vi "FM_RTL-SDR_RX - V4-Script1.vi"() -> ()   [LabVIEW 2013]
uses:
  <vilib>/sound2/lvsound2.llb/Sound Data Format.ctl
  <vilib>/Analysis/2dsp.llb/Rational Resample (single channel, DBL).vi
  <vilib>/sound2/lvsound2.llb/Sound Output Write (DBL Single).vi
  <instrlib>/rtlsdr/rtlsdr.lvlib
  <vilib>/Analysis/NI_AALPro.lvlib
panel:
  in  "Device index":u32
  out "Samples Acquired":u32
  out "# elements in queue":i32
  out "DevRefnum":u64
  out "XY Graph":cluster{dbl[], dbl[]}(graph)
  out "error out":errorcluster
  in  "sound format":T1={"sample rate (S/s)"=44100.0, "number of channels"=1, "bits per sample"=16}
  in  "stop":bool
  in  "Center frequency":u32=104300000
  in  "IQ rate":u32=286650
  out "error out":errorcluster
  # "FM Receiver"
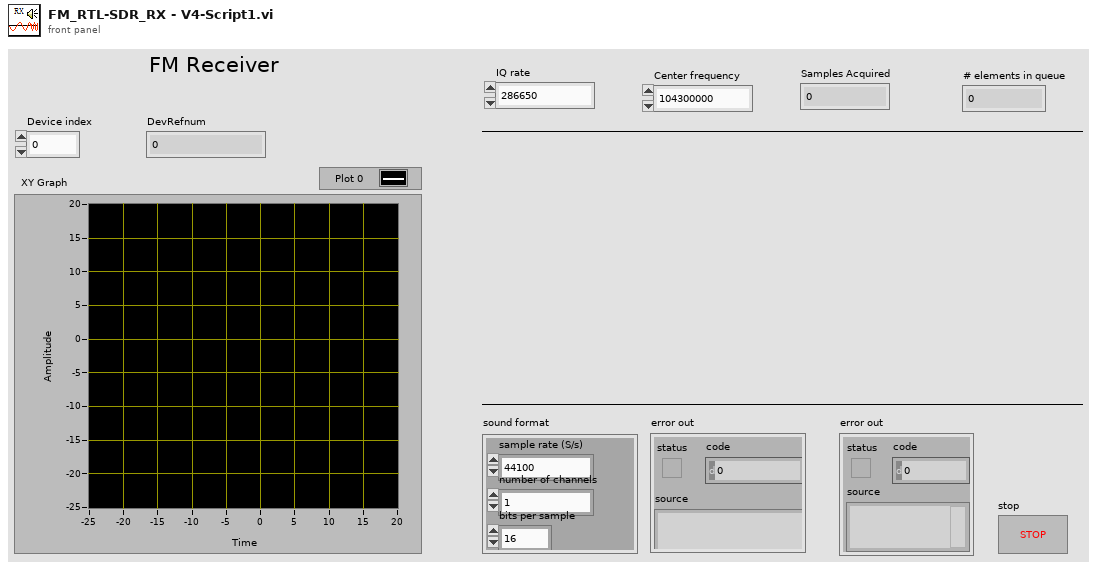
[diagram p1: front panel]
types:
  T1 = typedef "Sound Data Format.ctl" = cluster{"sample rate (S/s)":dbl, "number of channels":i32, "bits per sample":i32}
  T2 = typedef "Sound Output Task ID.ctl" = u32
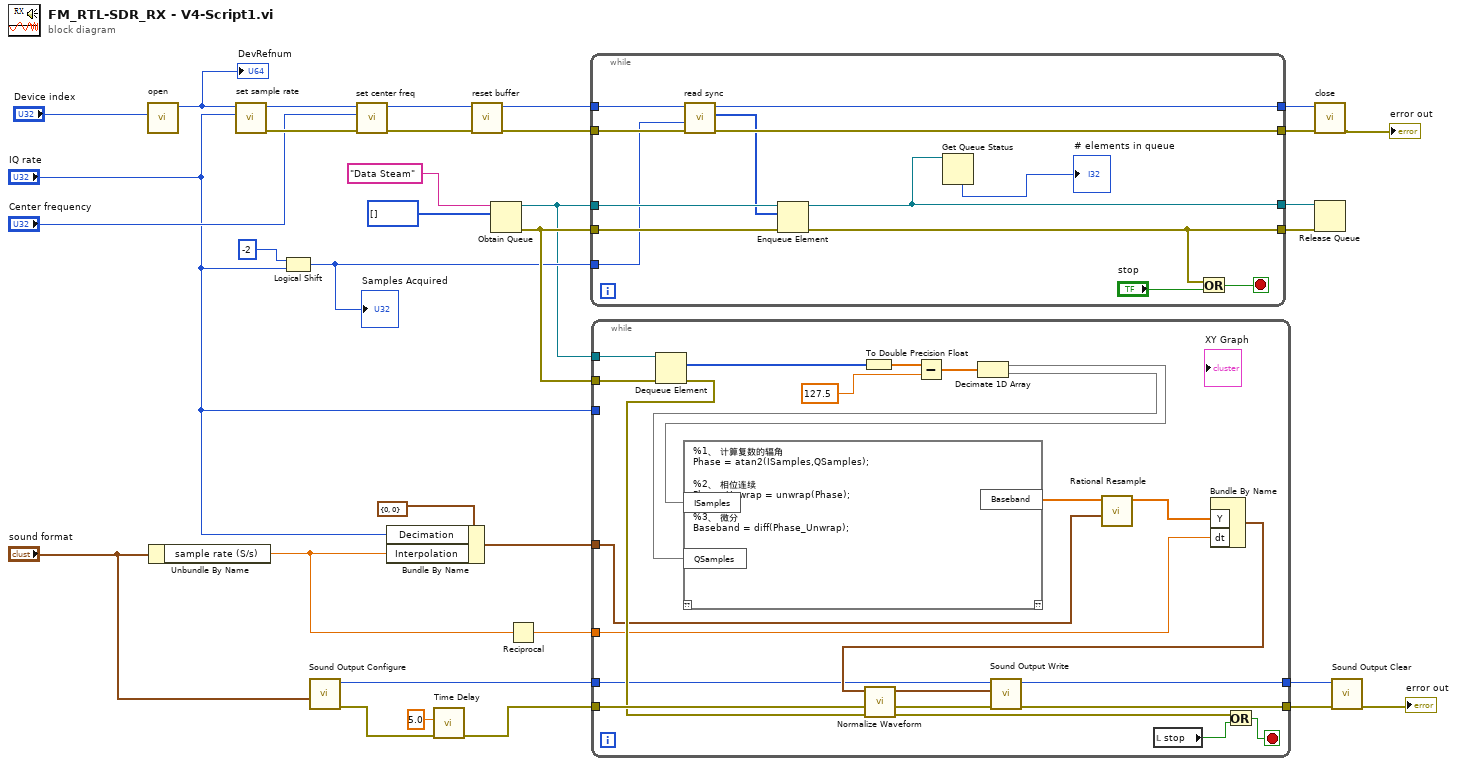
[diagram p0: block diagram]
diagram:
  n1 = call <instrlib>:"open.vi"("index"="Device index") -> ("DevRefnum"=w26:u64)  [unwired: 9 in, 1 out]
  "DevRefnum" <- w26
  n2 = Unbundle By Name("sound format") -> ("sample rate (S/s)"=w1:dbl)
  n3 = call <instrlib>:"set sample rate.vi"("rate"="IQ rate", "DevRefnum"=w26) -> ("error out"=w28:errorcluster, "DevRefnum"=w30:u64)  [unwired: 7 in, 1 out]
  n4 = Logical Shift(y=i16 -2, x="IQ rate") -> (x << y=w4:u32)
  "Samples Acquired" <- w4
  n5 = call <vilib>:"Sound Output Configure.vi"("sound format"="sound format") -> ("error out"=w8:errorcluster, "task ID"=w18:T2)  [unwired: 9 in]
  n6 = call <instrlib>:"set center freq.vi"("error in (no error)"=w28, "freq"="Center frequency", "DevRefnum"=w30) -> ("error out"=w27:errorcluster, "DevRefnum"=w29:u64)  [unwired: 6 in, 1 out]
  n7 = Bundle By Name(cluster=cluster{"Interpolation":i32, "Decimation":i32} {"Interpolation"=0, "Decimation"=0}, "Decimation"="IQ rate", "Interpolation"=w1) -> (w10:cluster{"Interpolation":i32, "Decimation":i32})
  n8 = call "Time Delay"("error in (no error)"=w8, "Delay Time (s)"=5.0) -> ("error out"=w9:errorcluster)  [unwired: 9 in]
  n9 = call <instrlib>:"reset buffer.vi"("error in (no error)"=w27, "DevRefnum"=w29) -> ("error out"=w23:errorcluster, "DevRefnum"=w24:u64)  [unwired: 8 in]
  n10 = Obtain Queue(name (unnamed)="Data Steam", element data type=u8[] [] ("buf 2")) -> (queue out=w3:refnum<queue>, error out=w5:errorcluster)  [unwired: 3 in, 1 out]
  n11 = Reciprocal(x=w1) -> (1/x=w11:dbl)
  n12 = while {
    tunnel: [w44] -> w21
    tunnel: w24 -> [w46]
    tunnel: w23 -> [w45]
    tunnel: [w43] -> w20
    tunnel: w4 -> [w34]
    tunnel: w3 -> [w41]
    tunnel: [w40] -> w14
    tunnel: w5 -> [w39]
    tunnel: [w37] -> w13
    stop <- w35 stop-if-true
    n13 = call <instrlib>:"read sync.vi"("error in (no error)"=w45, "len"=w34, "DevRefnum"=w46) -> ("error out"=w43:errorcluster, "buf 2"=w38:u8[], "DevRefnum"=w44:u64)  [unwired: 6 in]
    n14 = Enqueue Element(queue=w41, element=w38, error in (no error)=w39) -> (queue out=w40:refnum<queue>, error out=w37:errorcluster)  [unwired: 1 in, 1 out]
    n15 = Get Queue Status(queue=w40) -> (# elements in queue=→"# elements in queue":i32)  [unwired: 2 in, 7 out]
    n16 = Or(x=w37, y="stop") -> (x .or. y?=w35:bool)
  }
  n17 = while {
    tunnel: w18 -> [w52]
    tunnel: [w64] -> w17
    tunnel: [w63] -> w16
    tunnel: w9 -> [w65]
    tunnel: w3 -> [w62]
    tunnel: w11 -> [w53]
    tunnel: w10 -> [w48]
    tunnel: w5 -> [w58]
    tunnel: "IQ rate" -> [_]
    stop <- w54 stop-if-true
    n18 = Dequeue Element(queue=w62, error in (no error)=w58) -> (element=w61:u8[], error out=w57:errorcluster)  [unwired: 1 in, 2 out]
    n19 = To Double Precision Float(number=w61) -> (double precision float=w68:dbl[])
    n20 = Subtract(x=w68, y=127.5) -> (x-y=w66:dbl[])
    n21 = Decimate 1D Array "Decimate 1D Array"(w66) -> (w51:dbl[], w50:dbl[])
    n22 = script code="%1、 计算复数的辐角\nPhase = atan2(ISamples,QSamples);\n\n%2、 相位连续\nPhase_Unwrap = unwrap(Phase);\n\n%3、 微分\nBaseband = diff(Phase_Unwrap);"("ISamples"=w51, "QSamples"=w50) -> ("Baseband"=w49:dbl[])  [unwired: 1 in, 1 out]
    n23 = call-poly <vilib>:"Rational Resample.vi"("resample factor"=w48, "X"=w49) -> ("Y"=w47:dbl[])  [unwired: 7 in, 2 out]
    n24 = local read "stop"() -> (w55:bool)
    n25 = Bundle By Name ("Build Waveform")("Y"=w47, "dt"=w53) -> (w59:waveform(dbl))  [unwired: 1 in]
    n26 = call <vilib>:"Normalize Waveform.vi"("error in (no error)"=w57, "waveform in"=w59) -> ("error out"=w56:errorcluster, "normalized waveform"=w60:waveform(dbl))  [unwired: 6 in, 2 out]
    n27 = call-poly <vilib>:"Sound Output Write.vi"("error in (no error)"=w65, "data"=w60, "task ID"=w52) -> ("error out"=w63:errorcluster, "task ID out"=w64:T2)  [unwired: 7 in]
    n28 = Or(x=w56, y=w55) -> (x .or. y?=w54:bool)
  }
  n29 = call <instrlib>:"close.vi"("error in (no error)"=w20, "DevRefnum"=w21) -> ("error out"=→"error out":errorcluster)  [unwired: 8 in, 1 out]
  n30 = Release Queue(queue=w14, error in (no error)=w13) -> ()  [unwired: 1 in, 3 out]
  n31 = call <vilib>:"Sound Output Clear.vi"("error in (no error)"=w16, "task ID"=w17) -> ("error out"=→"error out":errorcluster)  [unwired: 9 in]
